vi "commandQuantity.vi"(8 "error in (no error)":errorcluster, 11 "CommandQueue in":refnum<class "CommandQueue.lvclass">) -> (0 "error out":errorcluster, 1 "x > 0?":bool, 2 "quant":i32, 3 "CommandQueue out":refnum<class "CommandQueue.lvclass">)   [LabVIEW 2016, in "CommandQueue.lvclass"]
uses:
  CommandQueue.lvclass
  CommandQueue.lvclass/CommandQueue.ctl
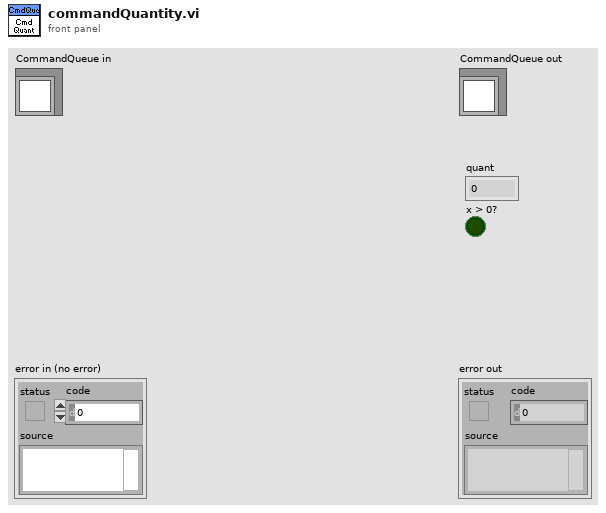
[diagram p1: front panel]
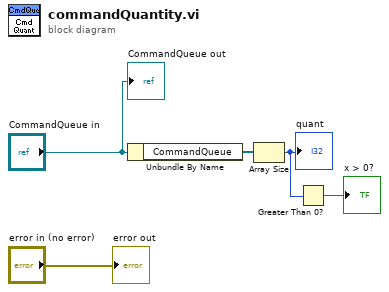
[diagram p0: block diagram]
diagram:
  n1 = Unbundle By Name("CommandQueue in") -> ("CommandQueue"=w3:refnum<class "Command.lvclass">[])
  n2 = Array Size(array=w3) -> (size(s)=w2:i32)
  "quant" <- w2
  n3 = Greater Than 0?(x=w2) -> (x > 0?=→"x > 0?":bool)
  "error out" <- "error in (no error)"
  "CommandQueue out" <- "CommandQueue in"
